vi "AttrMap-Merge.vi"(6 "If exist? Skip(T)/Overwrite(F)":bool=TRUE, 8 "error in (no error)":errorcluster, 10 "AttrMap B":T1, 11 "AttrMap A":T1) -> (0 "error out":errorcluster, 3 "AttrMap A after B->A":T1)   [LabVIEW 2019, in "lv-apt-json-file.lvlib"]
uses:
  lv-apt-json-file.lvlib
  Typedef/Def-AttrMap.ctl
  f16f814e-f0a0-47f4-ae2a-f78fd01390a2.vi
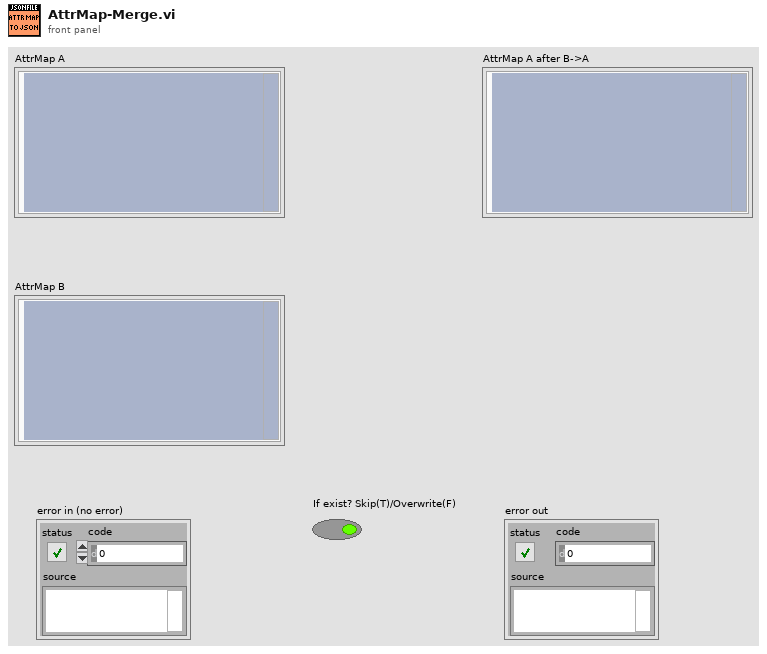
[diagram p1: front panel]
types:
  T1 = typedef "lv-apt-json-file.lvlib/Def-AttrMap.ctl" = cluster{"Map":variant}
  T2 = typedef "lv-apt-json-file.lvlib/Def-AttrMap -- NameMap.ctl" = map{string, string}
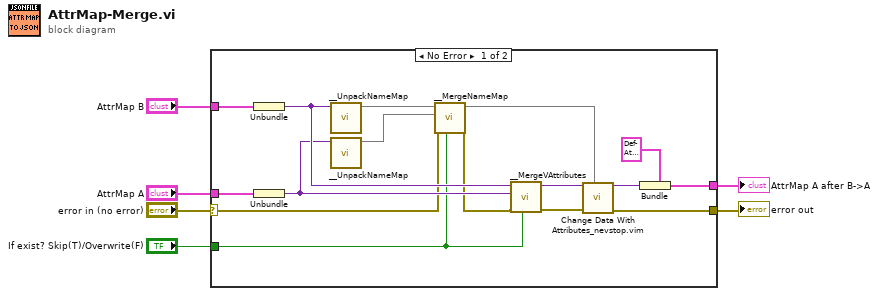
[diagram p0: block diagram]
diagram:
  n1 = case shown="No Error" "error in (no error)" {
    selector: "error in (no error)" -> [w8 w24]
    tunnel: "AttrMap A" -> [w22 w23]
    tunnel: "AttrMap B" -> [w21 _]
    tunnel: "If exist? Skip(T)/Overwrite(F)" -> [w11 _]
    tunnel: [w19 w24] -> w2
    tunnel: [w18 w23] -> w1
    frame No Error {
      n2 = Unbundle(w21) -> ("Map"=w13:variant)
      n3 = Unbundle(w22) -> ("Map"=w12:variant)
      n4 = call "__UnpackNameMap.vi"("Map"=w13) -> ("NameMap"=w16:T2)  [unwired: 10 in]
      n5 = call "__UnpackNameMap.vi"("Map"=w12) -> ("NameMap"=w15:T2)  [unwired: 10 in]
      n6 = call "__MergeNameMap.vi"("If exist? Skip(T)/Overwrite(F)"=w11, "error in (no error)"=w8, "NameMap B"=w15, "NameMap A"=w16) -> ("error out"=w7:errorcluster, "NameMap A after B->A"=w14:T2)  [unwired: 6 in]
      n7 = call "__MergeVAttributes.vi"("If exist? Skip(T)/Overwrite(F)"=w11, "error in (no error)"=w7, "VAttributes B"=w12, "VAttributes A"=w13) -> ("error out"=w9:errorcluster, "VAttributes A after B->A"=w10:variant)  [unwired: 6 in]
      n8 = call "Change Data With Attributes_nevstop.vim"("Data"=w14, "error in (no error)"=w9, "Variant in"=w10) -> ("error out"=w19:errorcluster, "Variant out"=w20:variant)  [unwired: 7 in]
      n9 = Bundle(cluster=T1 {"Map"=variant} ("AttrMap"), "Map"=w20) -> (w18:T1)
    }
    frame Error {
    }
  }
  "AttrMap A after B->A" <- w1
  "error out" <- w2
